vi "Quick Start.vi"() -> ()   [LabVIEW 2018]
uses:
  <vilib>/Platform/TimedLoop/XDataNode/timing_clust.ctl
  <vilib>/Platform/TimedLoop/XDataNode/nitl_modes.ctl
  <vilib>/Platform/TimedLoop/XDataNode/wakeup.ctl
  <extravilib>/ChannelInstances/Tag-bool/Read With Abort.vi
  <extravilib>/ChannelInstances/Tag-a[.](dbl)/Read With Abort.vi
  <extravilib>/ChannelInstances/Tag-bool/Write With Abort.vi
  <extravilib>/ChannelInstances/Tag-a[.](dbl)/Write With Abort.vi
  <extravilib>/ChannelInstances/Tag-bool/Instantiate.vi
  <extravilib>/ChannelInstances/Tag-bool/Endpoint.vi
  <extravilib>/ChannelInstances/Tag-a[.](dbl)/Instantiate.vi
  <extravilib>/ChannelInstances/Tag-bool/EndpointRead.vi
  <extravilib>/ChannelInstances/Tag-a[.](dbl)/EndpointRead.vi
  <extravilib>/ChannelInstances/Tag-a[.](dbl)/Endpoint.vi
  <vilib>/Platform/TimedLoop/XDataNode/XDataNode.xnode
  <vilib>/vision/NI_Vision_Development_Module.lvlib
  <extravilib>/ChannelInstances/Tag-a[.](dbl).lvlib
  <extravilib>/ChannelInstances/Tag-bool.lvlib
  <vilib>/Platform/TimedLoop/XDataNode/XDNodeRunTimeDep.lvlib
panel:
  out "End-effector Trajectory":cluster{dbl[], dbl[]}[](graph)=[{[0.0, 0.0, 0.0, 0.0, 0.0, 0.0, 0.0, 0.0, 0.0, 0.0, 0.0, 0.0, 0.0, 0.0, 0.0, 0.0, 0.0, 0.0, 0.0, 0.0, 0.0, 0.0, 0.0, 0.0, 0.0, 0.0, 0.0, 0.0, 0.0, 0.0, 0.0, 0.0, 0.0, 0.0, 0.0, 0.0, 0.0, 0.0, 0.0, 0.0, 0.0, 0.0, 0.0, 0.0, 0.0, 0.0, 0.0, 0.0, 0.0, 0.0, 0.0, 0.0, 0.0, 0.0, 0.0, 0.0, 0.0, 0.0, 0.0, 0.0, 0.0, 0.0, 0.0, 0.0, 0.0, 0.0, 0.0, 0.0, 0.0, 0.0, 0.0, 0.0, 0.0, 0.0, 0.0, 0.0, 0.0, 0.0, 0.0, 0.0, 0.0, 0.0, 0.0, 0.0, 0.0, 0.0, 0.0, 0.0, 0.0, 0.0, 0.0, 0.0, 0.0, 0.0, 0.0, 0.0, 0.0, 0.0, 0.0, 0.0, 0.0, 0.0, 0.0, 0.0, 0.0, 0.0, 0.0, 0.0, 0.0, 0.0, 0.0, 0.0, 0.0, 0.0, 0.0, 0.0, 0.0, 0.0, 0.0, 0.0, 0.0, 0.0, 0.0, 0.0, 0.0, 0.0, 0.0, 0.0, 0.0, 0.0, 0.0, 0.0, 0.0, 0.0, 0.0, 0.0, 0.0, 0.0, 0.0, 0.0, 0.0, 0.0, 0.0, 0.0, 0.0, 0.0, 0.0, 0.0, 0.0, 0.0, 0.0, 0.0, 0.0, 0.0, 0.0, 0.0, 0.0, 0.0, 0.0, 0.0, 0.0, 0.0, 0.0, 0.0, 0.0, 0.0, 0.0, 0.0, 0.0, 0.0, 0.0, 0.0, 0.0, 0.0, 0.0, 0.0, 0.0, 0.0, 0.0, 0.0, 0.0, 0.0, 0.0, 0.0, 0.0, 0.0, 0.0, 0.0, 0.0, 0.0, 0.0, 0.0, 0.0, 0.0, 0.0, 0.0, 0.0, 0.0, 0.0, 0.0, 0.0, 0.0, 0.0, 0.0, 0.0, 0.0, 0.0, 0.0, 0.0, 0.0, 0.0, 0.0, 0.0, 0.0, 0.0, 0.0, 0.0, 0.0, 0.0, 0.0, 0.0, 0.0, 0.0, 0.0, 0.0, 0.0, 0.0, 0.0, 0.0, 0.0, 0.0, 0.0, 0.0, 0.0, 0.0, 0.0, 0.0, 0.0, 0.0, 0.0, 0.0, 0.0, 0.0, 0.0, 0.0, 0.0, 0.0, 0.0, 0.0, 0.0, 0.0, 0.0, 0.0, 0.0, 0.0, 0.0, 0.0, 0.0, 0.0, 0.0, 0.0, 0.0, 0.0, 0.0, 0.0, 0.0, 0.0, 0.0, 0.0, 0.0, 0.0, 0.0, 0.0, 0.0, 0.0, 0.0, 0.0, 0.0, 0.0, 0.0, 0.0, 0.0, 0.0, 0.0, 0.0, 0.0, 0.0, 0.0, 0.0, 0.0, 0.0, 0.0, 0.0, 0.0, 0.0, 0.0, 0.0, 0.0, 0.0, 0.0, 0.0, 0.0, 0.0, 0.0, 0.0, 0.0, 0.0, 0.0, 0.0, 0.0, 0.0, 0.0, 0.0, 0.0, 0.0, 0.0, 0.0, 0.0, 0.0, 0.0, 0.0, 0.0, 0.0, 0.0, 0.0, 0.0, 0.0, 0.0, 0.0, 0.0, 0.0, 0.0, 0.0, 0.0, 0.0, 0.0, 0.0, 0.0, 0.0, 0.0, 0.0, 0.0, 0.0, 0.0, 0.0, 0.0, 0.0, 0.0, 0.0, 0.0, 0.0, 0.0, 0.0, 0.0, 0.0, 0.0, 0.0, 0.0, 0.0, 0.0, 0.0, 0.0, 0.0, 0.0, 0.0, 0.0, 0.0, 0.0, 0.0, 0.0, 0.0, 0.0, 0.0, 0.0, 0.0, 0.0, 0.0, 0.0, 0.0, 0.0, 0.0, 0.0, 0.0, 0.0, 0.0, 0.0, 0.0, 0.0, 0.0, 0.0, 0.0, 0.0, 0.0, 0.0, 0.0, 0.0, 0.0, 0.0, 0.0, 0.0, 0.0, 0.0, 0.0, 0.0, 0.0, 0.0, 0.0, 0.0, 0.0, 0.0, 0.0, 0.0, 0.0, 0.0, 0.0, 0.0, 0.0, 0.0, 0.0, 0.0, 0.0, 0.0, 0.0, 0.0, 0.0, 0.0, 0.0, 0.0, 0.0, 0.0, 0.0, 0.0, 0.0, 0.0, 0.0, 0.0, 0.0, 0.0, 0.0, 0.0, 0.0, 0.0, 0.0, 0.0, 0.0, 0.0, 0.0, 0.0, 0.0, 0.0, 0.0, 0.0, 0.0, 0.0, 0.0, 0.0, 0.0, 0.0, 0.0, 0.0, 0.0, 0.0, 0.0, 0.0, 0.0, 0.0, 0.0, 0.0, 0.0, 0.0, 0.0, 0.0, 0.0, 0.0, 0.0, 0.0, 0.0, 0.0, 0.0, 0.0, 0.0, 0.0, 0.0, 0.0, 0.0, 0.0, 0.0, 0.0, 0.0, 0.0, 0.0, 0.0, 0.0, 0.0, 0.0, 0.0, 0.0, 0.0, 0.0, 0.0, 0.0, 0.0, 0.0, 0.0, 0.0, 0.0, 0.0, 0.0, 0.0, 0.0, 0.0, 0.0], [0.0, 0.0, 0.0, 0.0, 0.0, 0.0, 0.0, 0.0, 0.0, 0.0, 0.0, 0.0, 0.0, 0.0, 0.0, 0.0, 0.0, 0.0, 0.0, 0.0, 0.0, 0.0, 0.0, 0.0, 0.0, 0.0, 0.0, 0.0, 0.0, 0.0, 0.0, 0.0, 0.0, 0.0, 0.0, 0.0, 0.0, 0.0, 0.0, 0.0, 0.0, 0.0, 0.0, 0.0, 0.0, 0.0, 0.0, 0.0, 0.0, 0.0, 0.0, 0.0, 0.0, 0.0, 0.0, 0.0, 0.0, 0.0, 0.0, 0.0, 0.0, 0.0, 0.0, 0.0, 0.0, 0.0, 0.0, 0.0, 0.0, 0.0, 0.0, 0.0, 0.0, 0.0, 0.0, 0.0, 0.0, 0.0, 0.0, 0.0, 0.0, 0.0, 0.0, 0.0, 0.0, 0.0, 0.0, 0.0, 0.0, 0.0, 0.0, 0.0, 0.0, 0.0, 0.0, 0.0, 0.0, 0.0, 0.0, 0.0, 0.0, 0.0, 0.0, 0.0, 0.0, 0.0, 0.0, 0.0, 0.0, 0.0, 0.0, 0.0, 0.0, 0.0, 0.0, 0.0, 0.0, 0.0, 0.0, 0.0, 0.0, 0.0, 0.0, 0.0, 0.0, 0.0, 0.0, 0.0, 0.0, 0.0, 0.0, 0.0, 0.0, 0.0, 0.0, 0.0, 0.0, 0.0, 0.0, 0.0, 0.0, 0.0, 0.0, 0.0, 0.0, 0.0, 0.0, 0.0, 0.0, 0.0, 0.0, 0.0, 0.0, 0.0, 0.0, 0.0, 0.0, 0.0, 0.0, 0.0, 0.0, 0.0, 0.0, 0.0, 0.0, 0.0, 0.0, 0.0, 0.0, 0.0, 0.0, 0.0, 0.0, 0.0, 0.0, 0.0, 0.0, 0.0, 0.0, 0.0, 0.0, 0.0, 0.0, 0.0, 0.0, 0.0, 0.0, 0.0, 0.0, 0.0, 0.0, 0.0, 0.0, 0.0, 0.0, 0.0, 0.0, 0.0, 0.0, 0.0, 0.0, 0.0, 0.0, 0.0, 0.0, 0.0, 0.0, 0.0, 0.0, 0.0, 0.0, 0.0, 0.0, 0.0, 0.0, 0.0, 0.0, 0.0, 0.0, 0.0, 0.0, 0.0, 0.0, 0.0, 0.0, 0.0, 0.0, 0.0, 0.0, 0.0, 0.0, 0.0, 0.0, 0.0, 0.0, 0.0, 0.0, 0.0, 0.0, 0.0, 0.0, 0.0, 0.0, 0.0, 0.0, 0.0, 0.0, 0.0, 0.0, 0.0, 0.0, 0.0, 0.0, 0.0, 0.0, 0.0, 0.0, 0.0, 0.0, 0.0, 0.0, 0.0, 0.0, 0.0, 0.0, 0.0, 0.0, 0.0, 0.0, 0.0, 0.0, 0.0, 0.0, 0.0, 0.0, 0.0, 0.0, 0.0, 0.0, 0.0, 0.0, 0.0, 0.0, 0.0, 0.0, 0.0, 0.0, 0.0, 0.0, 0.0, 0.0, 0.0, 0.0, 0.0, 0.0, 0.0, 0.0, 0.0, 0.0, 0.0, 0.0, 0.0, 0.0, 0.0, 0.0, 0.0, 0.0, 0.0, 0.0, 0.0, 0.0, 0.0, 0.0, 0.0, 0.0, 0.0, 0.0, 0.0, 0.0, 0.0, 0.0, 0.0, 0.0, 0.0, 0.0, 0.0, 0.0, 0.0, 0.0, 0.0, 0.0, 0.0, 0.0, 0.0, 0.0, 0.0, 0.0, 0.0, 0.0, 0.0, 0.0, 0.0, 0.0, 0.0, 0.0, 0.0, 0.0, 0.0, 0.0, 0.0, 0.0, 0.0, 0.0, 0.0, 0.0, 0.0, 0.0, 0.0, 0.0, 0.0, 0.0, 0.0, 0.0, 0.0, 0.0, 0.0, 0.0, 0.0, 0.0, 0.0, 0.0, 0.0, 0.0, 0.0, 0.0, 0.0, 0.0, 0.0, 0.0, 0.0, 0.0, 0.0, 0.0, 0.0, 0.0, 0.0, 0.0, 0.0, 0.0, 0.0, 0.0, 0.0, 0.0, 0.0, 0.0, 0.0, 0.0, 0.0, 0.0, 0.0, 0.0, 0.0, 0.0, 0.0, 0.0, 0.0, 0.0, 0.0, 0.0, 0.0, 0.0, 0.0, 0.0, 0.0, 0.0, 0.0, 0.0, 0.0, 0.0, 0.0, 0.0, 0.0, 0.0, 0.0, 0.0, 0.0, 0.0, 0.0, 0.0, 0.0, 0.0, 0.0, 0.0, 0.0, 0.0, 0.0, 0.0, 0.0, 0.0, 0.0, 0.0, 0.0, 0.0, 0.0, 0.0, 0.0, 0.0, 0.0, 0.0, 0.0, 0.0, 0.0, 0.0, 0.0, 0.0, 0.0, 0.0, 0.0, 0.0, 0.0, 0.0, 0.0, 0.0, 0.0, 0.0, 0.0, 0.0, 0.0, 0.0, 0.0, 0.0, 0.0, 0.0, 0.0, 0.0, 0.0, 0.0, 0.0, 0.0, 0.0, 0.0, 0.0, 0.0, 0.0, 0.0, 0.0, 0.0, 0.0, 0.0, 0.0, 0.0, 0.0, 0.0, 0.0, 0.0, 0.0, 0.0, 0.0, 0.0, 0.0, 0.0, 0.0, 0.0, 0.0, 0.0, 0.0, 0.0, 0.0, 0.0, 0.0, 0.0, 0.0]}, {[4.299999999999953, 4.3099999999999525, 4.319999999999952, 4.329999999999952, 4.339999999999952, 4.349999999999952, 4.3599999999999515, 4.369999999999951, 4.379999999999951, 4.389999999999951, 4.399999999999951, 4.40999999999995, 4.41999999999995, 4.42999999999995, 4.43999999999995, 4.4499999999999496, 4.459999999999949, 4.469999999999949, 4.479999999999949, 4.489999999999949, 4.4999999999999485, 4.509999999999948, 4.519999999999948, 4.529999999999948, 4.539999999999948, 4.549999999999947, 4.559999999999947, 4.569999999999947, 4.579999999999947, 4.589999999999947, 4.599999999999946, 4.609999999999946, 4.619999999999946, 4.629999999999946, 4.6399999999999455, 4.649999999999945, 4.659999999999945, 4.669999999999945, 4.679999999999945, 4.689999999999944, 4.699999999999944, 4.709999999999944, 4.719999999999944, 4.729999999999944, 4.739999999999943, 4.749999999999943, 4.759999999999943, 4.769999999999943, 4.7799999999999425, 4.789999999999942, 4.799999999999942, 4.809999999999942, 4.819999999999942, 4.8299999999999415, 4.839999999999941, 4.849999999999941, 4.859999999999941, 4.869999999999941, 4.87999999999994, 4.88999999999994, 4.89999999999994, 4.90999999999994, 4.9199999999999395, 4.929999999999939, 4.939999999999939, 4.949999999999939, 4.959999999999939, 4.9699999999999385, 4.979999999999938, 4.989999999999938, 4.999999999999938, 5.009999999999938, 5.019999999999937, 5.029999999999937, 5.039999999999937, 5.049999999999937, 5.0599999999999365, 5.069999999999936, 5.079999999999936, 5.089999999999936, 5.099999999999936, 5.1099999999999355, 5.119999999999935, 5.129999999999935, 5.139999999999935, 5.149999999999935, 5.159999999999934, 5.169999999999934, 5.179999999999934, 5.189999999999934, 5.199999999999934, 5.209999999999933, 5.219999999999933, 5.229999999999933, 5.239999999999933, 5.2499999999999325, 5.259999999999932, 5.269999999999932, 5.279999999999932, 5.289999999999932, 5.299999999999931, 5.309999999999931, 5.319999999999931, 5.329999999999931, 5.339999999999931, 5.34999999999993, 5.35999999999993, 5.36999999999993, 5.37999999999993, 5.3899999999999295, 5.399999999999929, 5.409999999999929, 5.419999999999929, 5.429999999999929, 5.4399999999999284, 5.449999999999928, 5.459999999999928, 5.469999999999928, 5.479999999999928, 5.489999999999927, 5.499999999999927, 5.509999999999927, 5.519999999999927, 5.5299999999999265, 5.539999999999926, 5.549999999999926, 5.559999999999926, 5.569999999999926, 5.5799999999999255, 5.589999999999925, 5.599999999999925, 5.609999999999925, 5.619999999999925, 5.629999999999924, 5.639999999999924, 5.649999999999924, 5.659999999999924, 5.6699999999999235, 5.679999999999923, 5.689999999999923, 5.699999999999923, 5.709999999999923, 5.7199999999999225, 5.729999999999922, 5.739999999999922, 5.749999999999922, 5.759999999999922, 5.769999999999921, 5.779999999999921, 5.789999999999921, 5.799999999999921, 5.809999999999921, 5.81999999999992, 5.82999999999992, 5.83999999999992, 5.84999999999992, 5.8599999999999195, 5.869999999999919, 5.879999999999919, 5.889999999999919, 5.899999999999919, 5.909999999999918, 5.919999999999918, 5.929999999999918, 5.939999999999918, 5.949999999999918, 5.959999999999917, 5.969999999999917, 5.979999999999917, 5.989999999999917, 5.9999999999999165, 6.009999999999916, 6.019999999999916, 6.029999999999916, 6.039999999999916, 6.0499999999999154, 6.059999999999915, 6.069999999999915, 6.079999999999915, 6.089999999999915, 6.099999999999914, 6.109999999999914, 6.119999999999914, 6.129999999999914, 6.1399999999999135, 6.149999999999913, 6.159999999999913, 6.169999999999913, 6.179999999999913, 6.1899999999999125, 6.199999999999912, 6.209999999999912, 6.219999999999912, 6.229999999999912, 6.239999999999911, 6.249999999999911, 6.259999999999911, 6.269999999999911, 6.2799999999999105, 6.28999999999991, 6.29999999999991, 6.30999999999991, 6.31999999999991, 6.3299999999999095, 6.339999999999909, 6.349999999999909, 6.359999999999909, 6.369999999999909, 6.379999999999908, 6.389999999999908, 6.399999999999908, 6.409999999999908, 6.419999999999908, 6.429999999999907, 6.439999999999907, 6.449999999999907, 6.459999999999907, 6.4699999999999065, 6.479999999999906, 6.489999999999906, 6.499999999999906, 6.509999999999906, 6.519999999999905, 6.529999999999905, 6.539999999999905, 6.549999999999905, 6.559999999999905, 6.569999999999904, 6.579999999999904, 6.589999999999904, 6.599999999999904, 6.6099999999999035, 6.619999999999903, 6.629999999999903, 6.639999999999903, 6.649999999999903, 6.659999999999902, 6.669999999999902, 6.679999999999902, 6.689999999999902, 6.699999999999902, 6.709999999999901, 6.719999999999901, 6.729999999999901, 6.739999999999901, 6.7499999999999005, 6.7599999999999, 6.7699999999999, 6.7799999999999, 6.7899999999999, 6.7999999999998995, 6.809999999999899, 6.819999999999899, 6.829999999999899, 6.839999999999899, 6.849999999999898, 6.859999999999898, 6.869999999999898, 6.879999999999898, 6.8899999999998975, 6.899999999999897, 6.909999999999897, 6.919999999999897, 6.929999999999897, 6.9399999999998965, 6.949999999999896, 6.959999999999896, 6.969999999999896, 6.979999999999896, 6.989999999999895, 6.999999999999895, 7.009999999999895, 7.019999999999895, 7.0299999999998946, 7.039999999999894, 7.049999999999894, 7.059999999999894, 7.069999999999894, 7.0799999999998935, 7.089999999999893, 7.099999999999893, 7.109999999999893, 7.119999999999893, 7.129999999999892, 7.139999999999892, 7.149999999999892, 7.159999999999892, 7.169999999999892, 7.179999999999891, 7.189999999999891, 7.199999999999891, 7.209999999999891, 7.2199999999998905, 7.22999999999989, 7.23999999999989, 7.24999999999989, 7.25999999999989, 7.269999999999889, 7.279999999999889, 7.289999999999889, 7.299999999999889, 7.309999999999889, 7.319999999999888, 7.329999999999888, 7.339999999999888, 7.349999999999888, 7.3599999999998875, 7.369999999999887, 7.379999999999887, 7.389999999999887, 7.399999999999887, 7.4099999999998865, 7.419999999999886, 7.429999999999886, 7.439999999999886, 7.449999999999886, 7.459999999999885, 7.469999999999885, 7.479999999999885, 7.489999999999885, 7.4999999999998845, 7.509999999999884, 7.519999999999884, 7.529999999999884, 7.539999999999884, 7.5499999999998835, 7.559999999999883, 7.569999999999883, 7.579999999999883, 7.589999999999883, 7.599999999999882, 7.609999999999882, 7.619999999999882, 7.629999999999882, 7.6399999999998816, 7.649999999999881, 7.659999999999881, 7.669999999999881, 7.679999999999881, 7.6899999999998805, 7.69999999999988, 7.70999999999988, 7.71999999999988, 7.72999999999988, 7.739999999999879, 7.749999999999879, 7.759999999999879, 7.769999999999879, 7.779999999999879, 7.789999999999878, 7.799999999999878, 7.809999999999878, 7.819999999999878, 7.8299999999998775, 7.839999999999877, 7.849999999999877, 7.859999999999877, 7.869999999999877, 7.879999999999876, 7.889999999999876, 7.899999999999876, 7.909999999999876, 7.919999999999876, 7.929999999999875, 7.939999999999875, 7.949999999999875, 7.959999999999875, 7.9699999999998745, 7.979999999999874, 7.989999999999874, 7.999999999999874, 8.009999999999874, 8.019999999999873, 8.029999999999873, 8.039999999999873, 8.049999999999873, 8.059999999999873, 8.069999999999872, 8.079999999999872, 8.089999999999872, 8.099999999999872, 8.109999999999872, 8.119999999999871, 8.129999999999871, 8.139999999999871, 8.14999999999987, 8.15999999999987, 8.16999999999987, 8.17999999999987, 8.18999999999987, 8.19999999999987, 8.20999999999987, 8.21999999999987, 8.229999999999869, 8.239999999999869, 8.249999999999869, 8.259999999999868, 8.269999999999868, 8.279999999999868, 8.289999999999868, 8.299999999999867, 8.309999999999867, 8.319999999999867, 8.329999999999867, 8.339999999999867, 8.349999999999866, 8.359999999999866, 8.369999999999866, 8.379999999999866, 8.389999999999866, 8.399999999999865, 8.409999999999865, 8.419999999999865, 8.429999999999865, 8.439999999999864, 8.449999999999864, 8.459999999999864, 8.469999999999864, 8.479999999999864, 8.489999999999863, 8.499999999999863, 8.509999999999863, 8.519999999999863, 8.529999999999863, 8.539999999999862, 8.549999999999862, 8.559999999999862, 8.569999999999862, 8.579999999999862, 8.589999999999861, 8.599999999999861, 8.60999999999986, 8.61999999999986, 8.62999999999986, 8.63999999999986, 8.64999999999986, 8.65999999999986, 8.66999999999986, 8.67999999999986, 8.68999999999986, 8.699999999999859, 8.709999999999859, 8.719999999999859, 8.729999999999858, 8.739999999999858, 8.749999999999858, 8.759999999999858, 8.769999999999857, 8.779999999999857, 8.789999999999857, 8.799999999999857, 8.809999999999857, 8.819999999999856, 8.829999999999856, 8.839999999999856, 8.849999999999856, 8.859999999999856, 8.869999999999855, 8.879999999999855, 8.889999999999855, 8.899999999999855, 8.909999999999854, 8.919999999999854, 8.929999999999854, 8.939999999999854, 8.949999999999854, 8.959999999999853, 8.969999999999853, 8.979999999999853, 8.989999999999853, 8.999999999999853, 9.009999999999852, 9.019999999999852, 9.019999999999852, 9.019999999999852, 9.019999999999852, 9.019999999999852, 9.019999999999852, 9.019999999999852, 9.019999999999852, 9.019999999999852, 9.019999999999852, 9.019999999999852, 9.019999999999852, 9.019999999999852, 9.019999999999852, 9.019999999999852, 9.019999999999852, 9.019999999999852, 9.019999999999852, 9.019999999999852, 9.019999999999852, 9.019999999999852, 9.019999999999852, 9.019999999999852, 9.019999999999852, 9.019999999999852, 9.019999999999852, 9.019999999999852, 9.019999999999852, 9.019999999999852, 9.019999999999852, 9.019999999999852, 9.019999999999852, 9.019999999999852, 9.019999999999852, 9.019999999999852, 9.019999999999852, 9.019999999999852, 9.019999999999852, 9.019999999999852, 9.019999999999852], [6.780000000000175, 6.780000000000175, 6.780000000000175, 6.780000000000175, 6.780000000000175, 6.780000000000175, 6.780000000000175, 6.780000000000175, 6.780000000000175, 6.780000000000175, 6.780000000000175, 6.780000000000175, 6.780000000000175, 6.780000000000175, 6.780000000000175, 6.780000000000175, 6.780000000000175, 6.780000000000175, 6.780000000000175, 6.780000000000175, 6.780000000000175, 6.780000000000175, 6.780000000000175, 6.780000000000175, 6.780000000000175, 6.780000000000175, 6.780000000000175, 6.780000000000175, 6.780000000000175, 6.780000000000175, 6.780000000000175, 6.780000000000175, 6.780000000000175, 6.780000000000175, 6.780000000000175, 6.780000000000175, 6.780000000000175, 6.780000000000175, 6.780000000000175, 6.780000000000175, 6.780000000000175, 6.780000000000175, 6.780000000000175, 6.780000000000175, 6.780000000000175, 6.780000000000175, 6.780000000000175, 6.780000000000175, 6.780000000000175, 6.780000000000175, 6.780000000000175, 6.780000000000175, 6.780000000000175, 6.780000000000175, 6.780000000000175, 6.780000000000175, 6.780000000000175, 6.780000000000175, 6.780000000000175, 6.780000000000175, 6.780000000000175, 6.780000000000175, 6.780000000000175, 6.780000000000175, 6.780000000000175, 6.780000000000175, 6.780000000000175, 6.780000000000175, 6.780000000000175, 6.780000000000175, 6.780000000000175, 6.780000000000175, 6.780000000000175, 6.780000000000175, 6.780000000000175, 6.780000000000175, 6.780000000000175, 6.780000000000175, 6.780000000000175, 6.780000000000175, 6.780000000000175, 6.780000000000175, 6.780000000000175, 6.780000000000175, 6.780000000000175, 6.780000000000175, 6.780000000000175, 6.780000000000175, 6.780000000000175, 6.780000000000175, 6.780000000000175, 6.780000000000175, 6.780000000000175, 6.780000000000175, 6.780000000000175, 6.780000000000175, 6.780000000000175, 6.780000000000175, 6.780000000000175, 6.780000000000175, 6.780000000000175, 6.780000000000175, 6.780000000000175, 6.780000000000175, 6.780000000000175, 6.780000000000175, 6.780000000000175, 6.780000000000175, 6.780000000000175, 6.780000000000175, 6.780000000000175, 6.780000000000175, 6.780000000000175, 6.780000000000175, 6.780000000000175, 6.780000000000175, 6.780000000000175, 6.780000000000175, 6.780000000000175, 6.780000000000175, 6.780000000000175, 6.780000000000175, 6.780000000000175, 6.780000000000175, 6.780000000000175, 6.780000000000175, 6.780000000000175, 6.780000000000175, 6.780000000000175, 6.780000000000175, 6.780000000000175, 6.780000000000175, 6.780000000000175, 6.780000000000175, 6.780000000000175, 6.780000000000175, 6.780000000000175, 6.780000000000175, 6.780000000000175, 6.780000000000175, 6.780000000000175, 6.780000000000175, 6.780000000000175, 6.780000000000175, 6.780000000000175, 6.780000000000175, 6.780000000000175, 6.780000000000175, 6.780000000000175, 6.780000000000175, 6.780000000000175, 6.780000000000175, 6.780000000000175, 6.780000000000175, 6.780000000000175, 6.780000000000175, 6.780000000000175, 6.780000000000175, 6.780000000000175, 6.780000000000175, 6.780000000000175, 6.780000000000175, 6.780000000000175, 6.780000000000175, 6.780000000000175, 6.780000000000175, 6.780000000000175, 6.780000000000175, 6.780000000000175, 6.780000000000175, 6.780000000000175, 6.780000000000175, 6.780000000000175, 6.780000000000175, 6.780000000000175, 6.780000000000175, 6.780000000000175, 6.780000000000175, 6.780000000000175, 6.780000000000175, 6.780000000000175, 6.780000000000175, 6.780000000000175, 6.780000000000175, 6.780000000000175, 6.780000000000175, 6.780000000000175, 6.780000000000175, 6.780000000000175, 6.780000000000175, 6.780000000000175, 6.780000000000175, 6.780000000000175, 6.780000000000175, 6.780000000000175, 6.780000000000175, 6.780000000000175, 6.780000000000175, 6.780000000000175, 6.780000000000175, 6.780000000000175, 6.780000000000175, 6.780000000000175, 6.780000000000175, 6.780000000000175, 6.780000000000175, 6.780000000000175, 6.780000000000175, 6.780000000000175, 6.780000000000175, 6.780000000000175, 6.780000000000175, 6.780000000000175, 6.780000000000175, 6.780000000000175, 6.780000000000175, 6.780000000000175, 6.780000000000175, 6.780000000000175, 6.780000000000175, 6.780000000000175, 6.780000000000175, 6.780000000000175, 6.780000000000175, 6.780000000000175, 6.780000000000175, 6.780000000000175, 6.780000000000175, 6.780000000000175, 6.780000000000175, 6.780000000000175, 6.780000000000175, 6.780000000000175, 6.780000000000175, 6.780000000000175, 6.780000000000175, 6.780000000000175, 6.780000000000175, 6.780000000000175, 6.780000000000175, 6.780000000000175, 6.780000000000175, 6.780000000000175, 6.780000000000175, 6.780000000000175, 6.780000000000175, 6.780000000000175, 6.780000000000175, 6.780000000000175, 6.780000000000175, 6.780000000000175, 6.780000000000175, 6.780000000000175, 6.780000000000175, 6.780000000000175, 6.780000000000175, 6.780000000000175, 6.780000000000175, 6.780000000000175, 6.780000000000175, 6.780000000000175, 6.780000000000175, 6.780000000000175, 6.780000000000175, 6.780000000000175, 6.780000000000175, 6.780000000000175, 6.780000000000175, 6.780000000000175, 6.780000000000175, 6.780000000000175, 6.780000000000175, 6.780000000000175, 6.780000000000175, 6.780000000000175, 6.780000000000175, 6.780000000000175, 6.780000000000175, 6.780000000000175, 6.780000000000175, 6.780000000000175, 6.780000000000175, 6.780000000000175, 6.780000000000175, 6.780000000000175, 6.780000000000175, 6.780000000000175, 6.780000000000175, 6.780000000000175, 6.780000000000175, 6.780000000000175, 6.780000000000175, 6.780000000000175, 6.780000000000175, 6.780000000000175, 6.780000000000175, 6.780000000000175, 6.780000000000175, 6.780000000000175, 6.780000000000175, 6.780000000000175, 6.780000000000175, 6.780000000000175, 6.780000000000175, 6.780000000000175, 6.780000000000175, 6.780000000000175, 6.780000000000175, 6.780000000000175, 6.780000000000175, 6.780000000000175, 6.780000000000175, 6.780000000000175, 6.780000000000175, 6.780000000000175, 6.780000000000175, 6.780000000000175, 6.780000000000175, 6.780000000000175, 6.780000000000175, 6.780000000000175, 6.780000000000175, 6.780000000000175, 6.780000000000175, 6.780000000000175, 6.780000000000175, 6.780000000000175, 6.780000000000175, 6.780000000000175, 6.780000000000175, 6.780000000000175, 6.780000000000175, 6.780000000000175, 6.780000000000175, 6.780000000000175, 6.780000000000175, 6.780000000000175, 6.780000000000175, 6.780000000000175, 6.780000000000175, 6.780000000000175, 6.780000000000175, 6.780000000000175, 6.780000000000175, 6.780000000000175, 6.780000000000175, 6.780000000000175, 6.780000000000175, 6.780000000000175, 6.780000000000175, 6.780000000000175, 6.780000000000175, 6.780000000000175, 6.780000000000175, 6.780000000000175, 6.780000000000175, 6.780000000000175, 6.780000000000175, 6.780000000000175, 6.780000000000175, 6.780000000000175, 6.780000000000175, 6.780000000000175, 6.780000000000175, 6.780000000000175, 6.780000000000175, 6.780000000000175, 6.780000000000175, 6.780000000000175, 6.780000000000175, 6.780000000000175, 6.780000000000175, 6.780000000000175, 6.780000000000175, 6.780000000000175, 6.780000000000175, 6.780000000000175, 6.780000000000175, 6.780000000000175, 6.780000000000175, 6.780000000000175, 6.780000000000175, 6.780000000000175, 6.780000000000175, 6.780000000000175, 6.780000000000175, 6.780000000000175, 6.780000000000175, 6.780000000000175, 6.780000000000175, 6.780000000000175, 6.780000000000175, 6.780000000000175, 6.780000000000175, 6.780000000000175, 6.780000000000175, 6.780000000000175, 6.780000000000175, 6.780000000000175, 6.780000000000175, 6.780000000000175, 6.780000000000175, 6.780000000000175, 6.780000000000175, 6.780000000000175, 6.780000000000175, 6.780000000000175, 6.780000000000175, 6.780000000000175, 6.780000000000175, 6.780000000000175, 6.780000000000175, 6.780000000000175, 6.780000000000175, 6.780000000000175, 6.780000000000175, 6.780000000000175, 6.780000000000175, 6.780000000000175, 6.780000000000175, 6.780000000000175, 6.780000000000175, 6.780000000000175, 6.780000000000175, 6.780000000000175, 6.780000000000175, 6.780000000000175, 6.780000000000175, 6.780000000000175, 6.780000000000175, 6.780000000000175, 6.780000000000175, 6.780000000000175, 6.780000000000175, 6.780000000000175, 6.780000000000175, 6.780000000000175, 6.780000000000175, 6.780000000000175, 6.780000000000175, 6.780000000000175, 6.780000000000175, 6.780000000000175, 6.780000000000175, 6.780000000000175, 6.780000000000175, 6.780000000000175, 6.780000000000175, 6.780000000000175, 6.780000000000175, 6.780000000000175, 6.780000000000175, 6.780000000000175, 6.780000000000175, 6.780000000000175, 6.780000000000175, 6.780000000000175, 6.780000000000175, 6.780000000000175, 6.780000000000175, 6.780000000000175, 6.780000000000175, 6.780000000000175, 6.780000000000175, 6.780000000000175, 6.780000000000175, 6.780000000000175, 6.780000000000175, 6.780000000000175, 6.780000000000175, 6.780000000000175, 6.780000000000175, 6.780000000000175, 6.790000000000175, 6.800000000000175, 6.810000000000175, 6.820000000000174, 6.830000000000174, 6.840000000000174, 6.850000000000174, 6.8600000000001735, 6.870000000000173, 6.880000000000173, 6.890000000000173, 6.900000000000173, 6.9100000000001724, 6.920000000000172, 6.930000000000172, 6.940000000000172, 6.950000000000172, 6.960000000000171, 6.970000000000171, 6.980000000000171, 6.990000000000171, 7.0000000000001705, 7.01000000000017, 7.02000000000017, 7.03000000000017, 7.04000000000017, 7.0500000000001695, 7.060000000000169, 7.070000000000169, 7.080000000000169, 7.090000000000169, 7.100000000000168, 7.110000000000168, 7.120000000000168, 7.130000000000168, 7.1400000000001675, 7.150000000000167, 7.160000000000167, 7.170000000000167]}]
  in  "Enable Motion":bool=TRUE
  in  "Stop Button":bool
  out "# of Matches":i32
  out "Calibrated":bool
  out "Template":T1(plugin-control)
  out "Camera Image":T1(plugin-control)
  # "Mechatronic Systems Board"
  # "Quick Start"
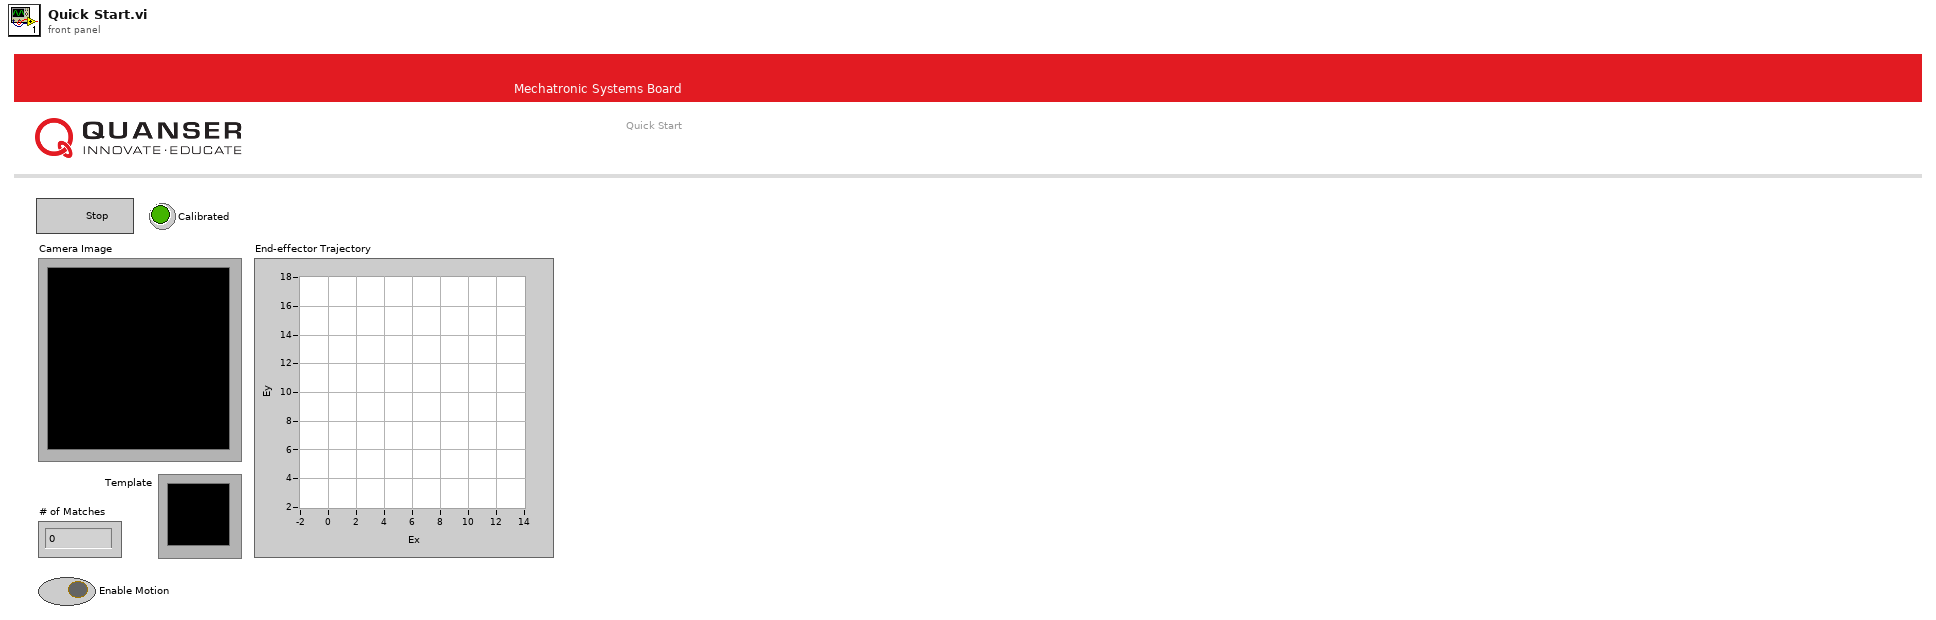
[diagram p1: front panel]
types:
  T1 = typedef "IMAQ Image.ctl" = refnum<image>
  T2 = cluster{"Algorithm":i32, "Number of Matches Requested":i32, "Minimum Match Score":sgl, "SubPixel Accuracy":bool, "Rotation Angle Ranges":cluster{"Start":sgl, "End":sgl}[], "Show Search Area":bool, "Show Result":bool}
  T3 = typedef "QNET MS IO Cluster.ctl" = cluster{"Error":errorcluster, "Encoder Calibration Values":i32[], "Update Calibration":bool, "JPEG Resolutions":u16, "Raw Resolutions":u16, "Image Mode":enum16{"RAW RGB", "RAW Gray Scale", "JPEG"}, "FPGA Ref":refnum<k20>}
  T4 = typedef "XDNodeRunTimeDep.lvlib/timing_clust.ctl" = cluster{"Expected End [f-1]":u64, "Actual End [f-1]":u64, "Finished Late? [f-1]":bool, "Expected End [i-1]":u64, "Actual End [i-1]":u64, "Finished Late? [i-1]":bool, "Expected Start [i]":u64, "Actual Start [i]":u64, "Expected Start [f]":u64, "Actual Start [f]":u64, "Source Name":string, "Structure Name":string, "Period":i64, "Deadline":i64, "Offset":i64, "Start":i64, "Priority":i32, "Timeout":i32, "Mode":T5, "Wakeup Reason":T6, "Error":errorcluster, "Source Type":string, "Secondary Source Type":string, "Global End Time":u64, "Global Start Time":u64, "Frame Duration":u64, "Iteration Duration":u64, "Assigned CPU":i32, "I/O Scan Engine Mode":u32}
  T5 = typedef "XDNodeRunTimeDep.lvlib/nitl_modes.ctl" = enum32{"No Change", "Process missed periods, maintain original phase", "Discard missed periods, maintain original phase", "Process missed periods, ignore original phase", "Discard missed periods, ignore original phase"}
  T6 = typedef "XDNodeRunTimeDep.lvlib/wakeup.ctl" = enum32{"Normal", "Aborted", "Asynchronous wakeup", "Timing source error", "Timed loop error", "Timeout"}
  T7 = typedef "Tag-bool.lvlib/))Channel.ctl" = refnum<queue>
  T8 = typedef "Tag-a[.](dbl).lvlib/))Channel.ctl" = refnum<queue>
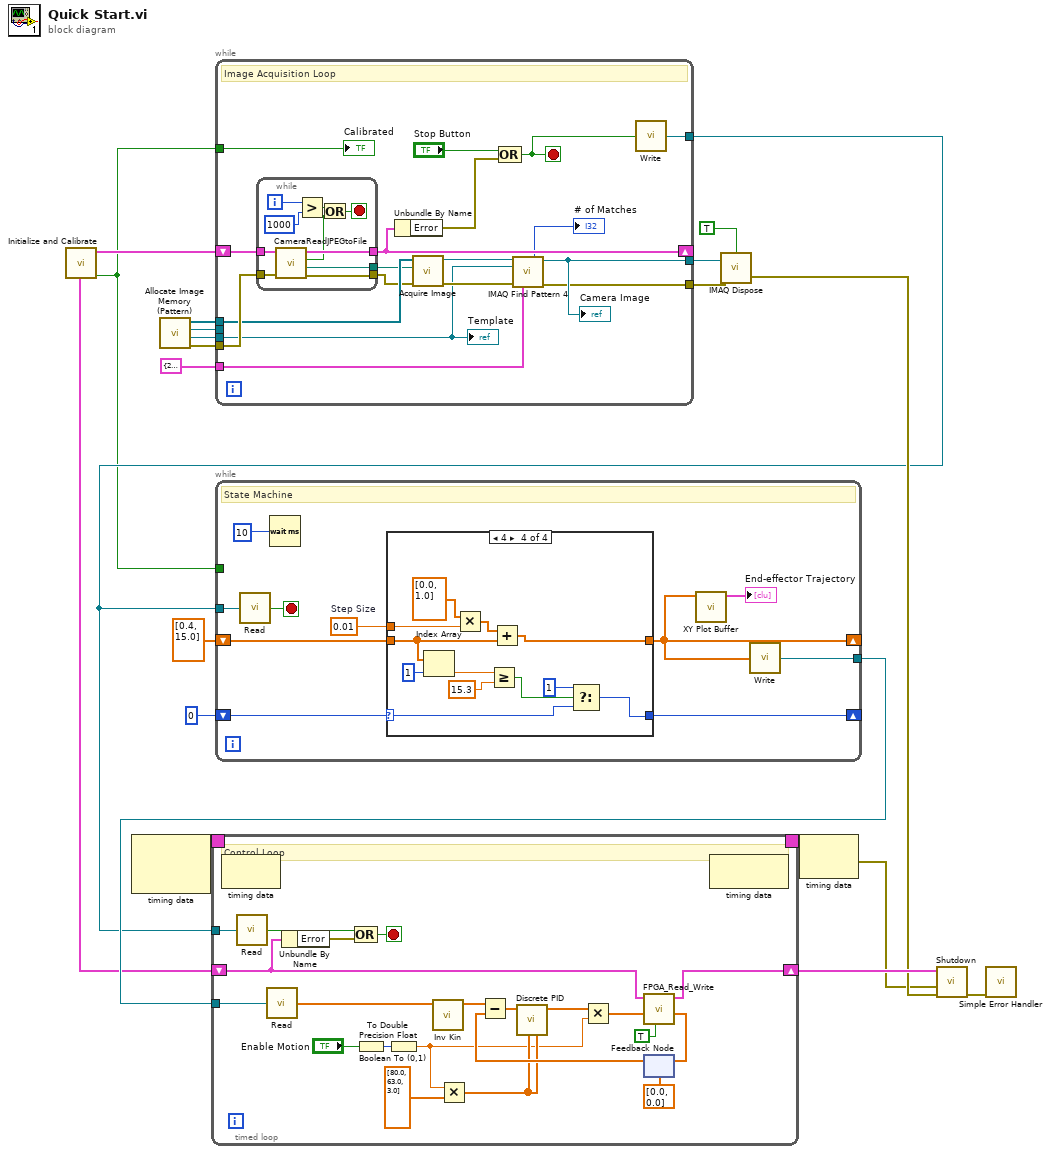
[diagram p0: block diagram]
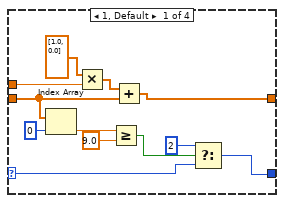
[diagram p2: hidden frame]
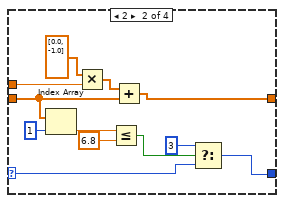
[diagram p3: hidden frame]
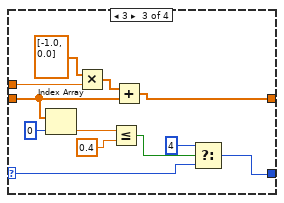
[diagram p4: hidden frame]
diagram:
  n1 = call "Initialize and Calibrate.vi"() -> ("Calibrated"=w1:bool, "IO Cluster"=w4:T3)  [unwired: 10 in]
  n2 = node-c288() -> (w16:T4)  [unwired: 2 in]
  n3 = call "Allocate Image Memory (Pattern).vi"() -> ("error out"=w20:errorcluster, "Template"=w17:T1, "Process Memory"=w18:T1, "Acquisition Memory"=w19:T1[])  [unwired: 8 in]
  n4 = while {
    tunnel: [w30] -> w9
    tunnel: [w33] -> w8
    tunnel: w20 -> [w37]
    tunnel: w19 -> [w36]
    tunnel: w18 -> [_]
    tunnel: w1 -> [w29]
    shift-right: [w28] -> _
    shift-left: w4 -> [w38]
    tunnel: w17 -> [w24]
    tunnel: [w23] -> w3
    tunnel: T2 {"Algorithm"=2, "Number of Matches Requested"=1, "Minimum Match Score"=800.0, "SubPixel Accuracy"=TRUE, "Rotation Angle Ranges"=[{"Start"=0.0, "End"=360.0}], "Show Search Area"=FALSE, "Show Result"=TRUE} ("Settings") -> [w22]
    stop <- w26 stop-if-true
    # "Image Acquisition Loop"
    n5 = while {
      tunnel: [w44] -> w35
      tunnel: w38 -> [w48]
      tunnel: [w47] -> w28
      tunnel: w37 -> [w45]
      tunnel: [w46] -> w32
      i -> [w40]
      stop <- w43 stop-if-true
      n6 = call "CameraReadJPEGtoFile.vi"("error in"=w45, "IO Cluster In"=w48) -> ("Error Out"=w46:errorcluster, "Image File"=w44:path, "New Image Data"=w39:bool, "IO Cluster Out"=w47:T3)  [unwired: 6 in]
      n7 = Greater?(x=w40, y=1000) -> (0:w42:bool)
      n8 = Or(x=w42, y=w39) -> (x .or. y?=w43:bool)
    }
    n9 = Unbundle By Name(w28) -> ("Error"=w27:errorcluster)
    n10 = call "Acquire Image.vi"("Error In"=w32, "File Path"=w35, "Acquisition Memory"=w36) -> ("Error Out"=w31:errorcluster, "Pre-processed Image"=w34:T1)  [unwired: 5 in, 2 out]
    n11 = Compound Arithmetic op=OR("Stop Button", w27) -> (w26:bool)
    n12 = call "IMAQ Find Pattern 4"("Image"=w34, "Template"=w24, "error in"=w31, "Settings"=w22) -> ("Number of Matches"=→"# of Matches":i32, "Image Out"=w33:T1, "error out"=w30:errorcluster)  [unwired: 5 in, 4 out]
    "Camera Image" <- w33
    n13 = call <extravilib>:"Write.vi"("element"=w26) -> ("channel"=w23:T7)  [unwired: 1 out]
    "Template" <- w24
    "Calibrated" <- w29
  }
  n14 = while {
    tunnel: [w58] -> w12
    tunnel: w3 -> [w57]
    shift-right: [w53] -> _
    shift-left: u32 0 ("millisecond multiple") -> [w51]
    shift-right: [w50] -> _
    shift-left: dbl[] [0.4, 15.0] ("appended array") -> [w55]
    tunnel: w1 -> [_]
    stop <- w56 stop-if-true
    w54 = 0.01  # Step Size
    # "State Machine"
    n15 = call <extravilib>:"Read.vi"("channel"=w57) -> ("element"=w56:bool)  [unwired: 1 in, 1 out]
    n16 = Wait (ms)(milliseconds to wait=u32 10 ("millisecond multiple")) -> ()  [unwired: 1 out]
    n17 = case shown="4" w51 {
      selector: w51 -> [w62 w73 w85 w97]
      tunnel: w55 -> [w66 w77 w89 w101]
      tunnel: [w67 w79 w91 w103] -> w50
      tunnel: w54 -> [w69 w81 w93 w105]
      tunnel: [w61 w72 w84 w96] -> w53
      frame 1, Default {
        n18 = Index Array(array=w66, index=0) -> (element=w65:dbl)
        n19 = Multiply(x=dbl[] [1.0, 0.0] ("appended array"), y=w69) -> (x*y=w70:dbl[])
        n20 = Greater Or Equal?(x=w65, y=9.0) -> (x >= y?=w63:bool)
        n21 = Add(x=w70, y=w66) -> (x+y=w67:dbl[])
        n22 = Select(t=u32 2, s=w63, f=w62) -> (s? t:f=w61:u32)
      }
      frame 2 {
        n23 = Index Array(array=w77, index=1) -> (element=w76:dbl)
        n24 = Multiply(x=dbl[] [0.0, -1.0] ("appended array"), y=w81) -> (x*y=w82:dbl[])
        n25 = Less Or Equal?(x=w76, y=6.8) -> (x <= y?=w74:bool)
        n26 = Add(x=w82, y=w77) -> (x+y=w79:dbl[])
        n27 = Select(t=u32 3, s=w74, f=w73) -> (s? t:f=w72:u32)
      }
      frame 3 {
        n28 = Index Array(array=w89, index=0) -> (element=w88:dbl)
        n29 = Multiply(x=dbl[] [-1.0, 0.0] ("appended array"), y=w93) -> (x*y=w94:dbl[])
        n30 = Less Or Equal?(x=w88, y=0.4) -> (x <= y?=w86:bool)
        n31 = Add(x=w94, y=w89) -> (x+y=w91:dbl[])
        n32 = Select(t=u32 4, s=w86, f=w85) -> (s? t:f=w84:u32)
      }
      frame 4 {
        n33 = Index Array(array=w101, index=1) -> (element=w100:dbl)
        n34 = Multiply(x=dbl[] [0.0, 1.0] ("appended array"), y=w105) -> (x*y=w106:dbl[])
        n35 = Greater Or Equal?(x=w100, y=15.3) -> (x >= y?=w98:bool)
        n36 = Add(x=w106, y=w101) -> (x+y=w103:dbl[])
        n37 = Select(t=u32 1, s=w98, f=w97) -> (s? t:f=w96:u32)
      }
    }
    n38 = call "XY Plot Buffer.vi"("Actual"=w50) -> ("Buffered Task Coordinates"=→"End-effector Trajectory":cluster{dbl[], dbl[]}[])  [unwired: 10 in]
    n39 = call <extravilib>:"Write.vi"("element"=w50) -> ("channel"=w58:T8)  [unwired: 1 out]
  }
  n40 = timed-loop {
    timing: w16 -> [_]
    timing-out: [_] -> w15
    shift-right: [w122] -> w7
    shift-left: w4 -> [w123]
    tunnel: w12 -> [w109]
    tunnel: w3 -> [w108]
    stop <- w117 stop-if-true
    # "Control Loop"
    n41 = node-c288() -> ()  [unwired: 1 in, 1 out]
    n42 = call <extravilib>:"Read.vi"("channel"=w108) -> ("element"=w107:bool)  [unwired: 1 in, 1 out]
    n43 = call <extravilib>:"Read.vi"("channel"=w109) -> ("element"=w126:dbl[])  [unwired: 1 in, 1 out]
    n44 = Unbundle By Name(w123) -> ("Error"=w127:errorcluster)
    n45 = Compound Arithmetic op=OR(w107, w127) -> (w117:bool)
    n46 = Boolean To (0,1)(Boolean="Enable Motion") -> (0, 1=w113:i16)
    n47 = To Double Precision Float(number=w113) -> (double precision float=w110:dbl)
    n48 = call "Inv Kin.vi"("Task Coordinates (cm)"=w126) -> ("Joint Coordinates (rad)"=w125:dbl[])  [unwired: 10 in]
    n49 = Multiply(x=w110, y=dbl[] [80.0, 63.0, 3.0] ("Joint Coordinates (rad)")) -> (x*y=w114:dbl[])
    n50 = feedback #1(dbl[] [0.0, 0.0] ("Joint Coordinates (rad)")) -> (w120:dbl[])
    n51 = Subtract(x=w125, y=w120) -> (x-y=w124:dbl[])
    n52 = call "Discrete PID.vi"("Gains Motor 1"=w114, "Gains Motor 0"=w114, "Error Array"=w124) -> ("Voltage"=w112:dbl[])  [unwired: 8 in]
    n53 = Multiply(x=w112, y=w110) -> (x*y=w111:dbl[])
    n54 = call "FPGA_Read_Write.vi"("Motors enabled?"=TRUE, "Commands"=w111, "IO Cluster In"=w123) -> ("Joint Coordinates (rad)"=w121:dbl[], "IO Cluster Out"=w122:T3)  [unwired: 5 in, 2 out]
    n55 = feedback-in #1(w121) -> ()
    n56 = node-c288() -> ()  [unwired: 1 in, 1 out]
  }
  n57 = call "IMAQ Dispose"("All Images? (No)"=TRUE, "Image"=w8, "error in (no error)"=w9) -> ("error out"=w6:errorcluster)  [unwired: 3 in]
  n58 = node-c288(w15) -> (w5:errorcluster)
  n59 = call "Shutdown.vi"("Image Processing Loop"=w6, "Manipulator Loop"=w5, "IO Cluster In"=w7) -> ("Error"=w10:errorcluster)  [unwired: 8 in]
  n60 = call <vilib>:"Simple Error Handler.vi"("error in (no error)"=w10) -> ()  [unwired: 4 in, 5 out]
